vi "Sub01_PixmapBin.vi"(8 "error in (no error)":errorcluster, 10 "path to PNG file":path, 11 "base path":path) -> (0 "error out 2":errorcluster, 3 "Image Disp":picture)   [LabVIEW 2019]
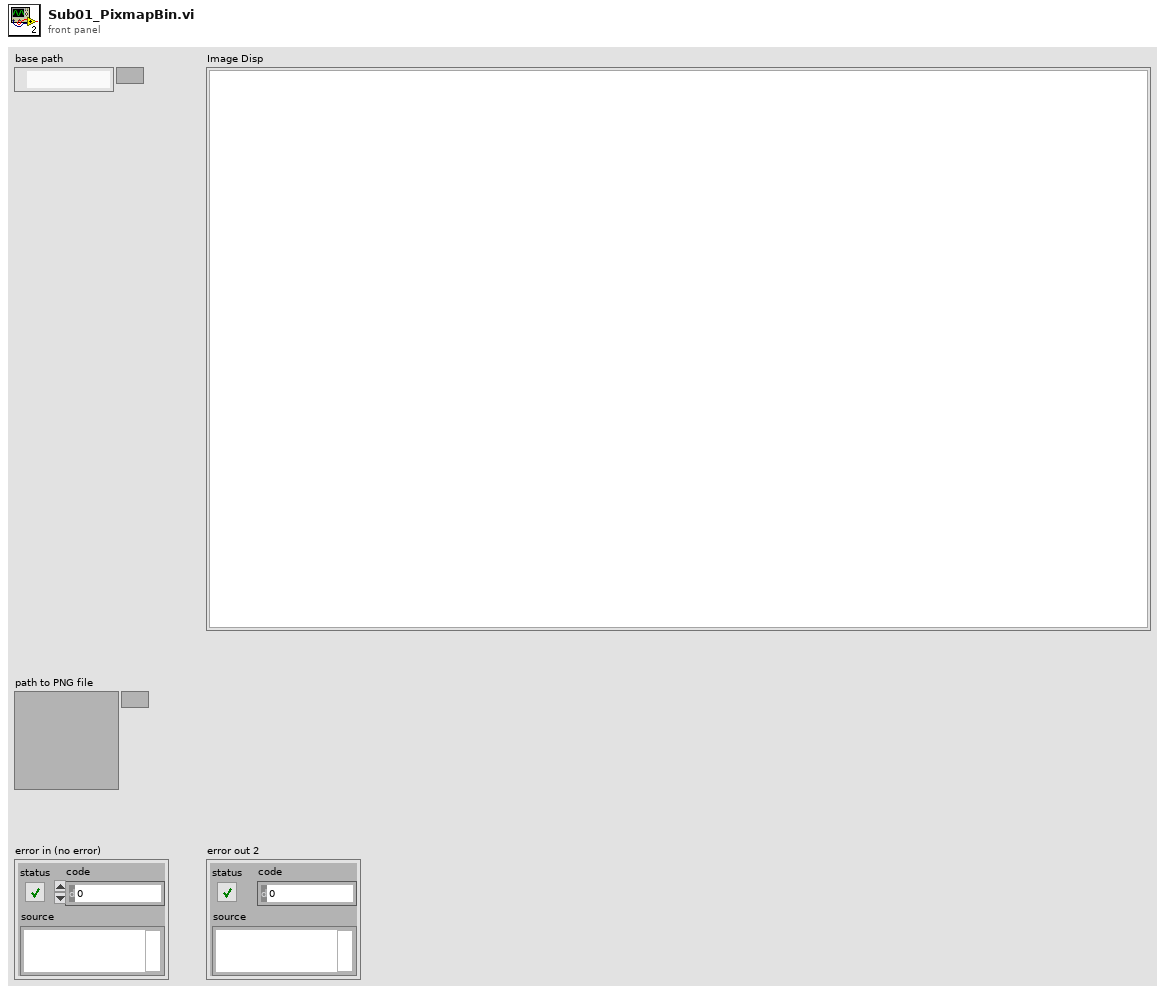
[diagram p1: front panel]
types:
  T1 = enum16{"big-endian, network order", "native, host order", "little-endian"}
  T2 = typedef "imagedata.ctl" = cluster{"image type":i32, "image depth":i32, "image":u8[], "mask":u8[], "colors":u32[], "Rectangle":cluster{"left":i16, "top":i16, "right":i16, "bottom":i16}}
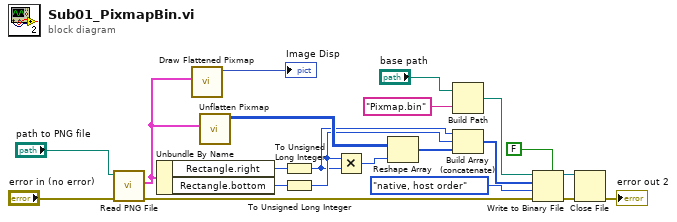
[diagram p0: block diagram]
diagram:
  n1 = call <vilib>:"Read PNG File.vi"("error in (no error)"="error in (no error)", "path to PNG file"="path to PNG file") -> ("error out"=w3:errorcluster, "image data"=w19:T2)  [unwired: 7 in, 1 out]
  n2 = Unbundle By Name(w19) -> ("Rectangle.right"=w15:i16, "Rectangle.bottom"=w16:i16)
  n3 = call <vilib>:"Draw Flattened Pixmap.vi"("image data"=w19) -> ("new picture"=→"Image Disp":picture)  [unwired: 8 in]
  n4 = call <vilib>:"Unflatten Pixmap.vi"("image data"=w19) -> ("24-bit pixmap"=w17:u32[][])  [unwired: 4 in, 6 out]
  n5 = To Unsigned Long Integer(number=w15) -> (unsigned 32bit integer=w12:u32)
  n6 = To Unsigned Long Integer(number=w16) -> (unsigned 32bit integer=w13:u32)
  n7 = Multiply(x=w13, y=w12) -> (x*y=w14:u32)
  n8 = Reshape Array(w17, w14) -> (w18:u32[])
  n9 = Build Path(base path="base path", name or relative path="Pixmap.bin" ("string")) -> (appended path=w6:path)
  n10 = Build Array (concatenate)(w12, w13, w18) -> (w2:u32[])
  n11 = Write to Binary File(file (use dialog)=w6, data=w2, error in=w3, 5:FALSE ("prepend array or string size? (T)"), 9:T1."native, host order" ("byte order (0:big-endian, network order)")) -> (refnum out=w9:refnum<file>, error out=w10:errorcluster)  [unwired: 1 in, 1 out]
  n12 = Close File(refnum=w9, error in=w10) -> (error out=→"error out 2":errorcluster)  [unwired: 1 out]
